vi "Noise Example VISA.vi"() -> ()   [LabVIEW 2012]
doc: "This example demonstrates how to use the various statistics VI's in the Analysis Library to generate common descriptive statistics quantities."
uses:
  <vilib>/Analysis/baseanly.llb/Unimode.vi
  <vilib>/Analysis/NI_AALPro.lvlib
  <vilib>/Analysis/NI_AALBase.lvlib
panel:
  in  "medie":i32=36
  out "Noise 2":dbl[](graph)
  out "Histogram 2":T1(graph)
  out "Mean 2":dbl=0.028574228286743178 format="%.2f"
  out "STD 2":dbl=0.9724758954834173 format="%.2f"
  out "Variance 2":dbl=0.028574228286743168 format="%.2f"
  out "Skewness 2":dbl=0.2146149630445097 format="%.2f"
  out "Kurtosis 2":dbl=2.530711352055369 format="%.2f"
  out "Mode 2":dbl=0.23823547363281233 format="%.2f"
  out "Mode":dbl=0.23823547363281233 format="%.2f"
  out "Kurtosis":dbl=2.530711352055369 format="%.2f"
  out "Skewness":dbl=0.2146149630445097 format="%.2f"
  out "Variance":dbl=0.028574228286743168 format="%.2f"
  out "STD":dbl=0.9724758954834173 format="%.2f"
  out "Mean":dbl=0.028574228286743178 format="%.2f"
  in  "Intervals":i32=100
  in  "Samples":i32=500
  out "Noise":dbl[](graph)
  out "Histogram":T1(graph)
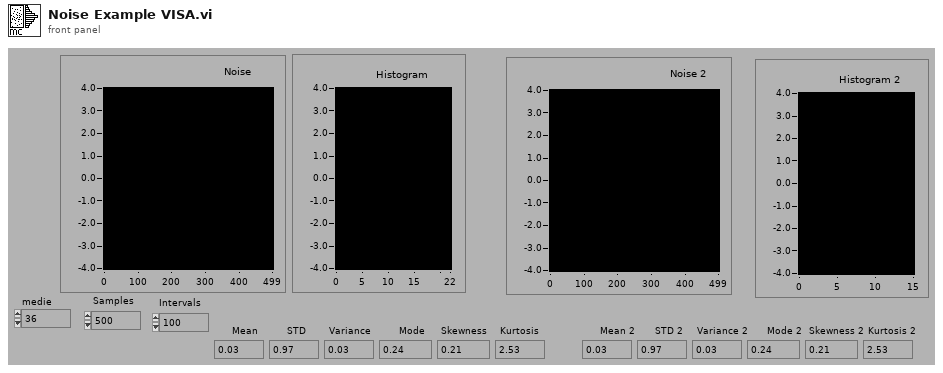
[diagram p1: front panel]
types:
  T1 = cluster{"Histogram: h(x)":i32[], "X Values":dbl[]}
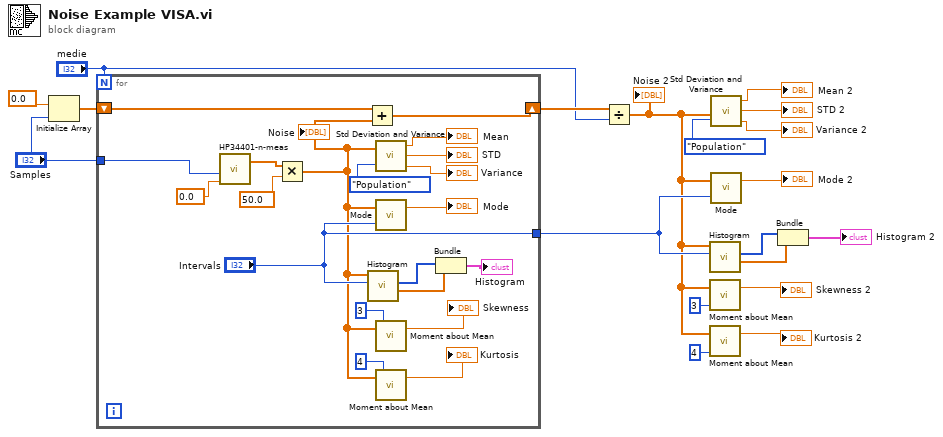
[diagram p0: block diagram]
diagram:
  n1 = Initialize Array(0.0 ("Element Data"), "Samples") -> (w1:dbl[])
  n2 = for {
    N: "medie" -> [_]
    tunnel: ["Intervals"] -> w7
    shift-right: [w26] -> w6
    shift-left: w1 -> [w25]
    tunnel: "Samples" -> [w24]
    n3 = call "HP34401-n-meas.vi"("Tc"=sgl 0.0, "N"=w24) -> ("Vet out"=w21:dbl[])  [unwired: 2 in, 1 out]
    n4 = Multiply(x=w21, y=50.0) -> (x*y=w20:dbl[])
    "Noise" <- w20
    n5 = Add(x=w25, y=w20) -> (x+y=w26:dbl[])
    n6 = call <vilib>:"Histogram.vi"("intervals"="Intervals", "X"=w20) -> ("X Values"=w39:dbl[], "Histogram: h(x)"=w38:i32[])  [unwired: 6 in, 2 out]
    n7 = call <vilib>:"Std Deviation and Variance.vi"("X"=w20, "Weighting (Sample)"=enum16{"Sample", "Population"}."Population") -> ("mean"=→"Mean":dbl, "standard deviation"=→"STD":dbl, "variance"=→"Variance":dbl)
    n8 = call-poly <vilib>:"Mode.vi"("intervals"="Intervals", "X"=w20) -> ("mode"=→"Mode":dbl)  [unwired: 1 out]
    n9 = call <vilib>:"Moment about Mean.vi"("order"=3, "X"=w20) -> ("moment"=→"Skewness":dbl)  [unwired: 1 out]
    n10 = call <vilib>:"Moment about Mean.vi"("order"=4, "X"=w20) -> ("moment"=→"Kurtosis":dbl)  [unwired: 1 out]
    n11 = Bundle("Histogram: h(x)"=w38, "X Values"=w39) -> (→"Histogram":T1)  [unwired: 1 in]
  }
  n12 = Divide(x=w6, y="medie") -> (x/y=w4:dbl[])
  "Noise 2" <- w4
  n13 = call <vilib>:"Histogram.vi"("intervals"=w7, "X"=w4) -> ("X Values"=w8:dbl[], "Histogram: h(x)"=w9:i32[])  [unwired: 6 in, 2 out]
  n14 = call <vilib>:"Moment about Mean.vi"("order"=3, "X"=w4) -> ("moment"=→"Skewness 2":dbl)  [unwired: 1 out]
  n15 = call <vilib>:"Moment about Mean.vi"("order"=4, "X"=w4) -> ("moment"=→"Kurtosis 2":dbl)  [unwired: 1 out]
  n16 = call <vilib>:"Std Deviation and Variance.vi"("X"=w4, "Weighting (Sample)"=enum16{"Sample", "Population"}."Population") -> ("mean"=→"Mean 2":dbl, "standard deviation"=→"STD 2":dbl, "variance"=→"Variance 2":dbl)
  n17 = call-poly <vilib>:"Mode.vi"("intervals"=w7, "X"=w4) -> ("mode"=→"Mode 2":dbl)  [unwired: 1 out]
  n18 = Bundle("Histogram: h(x)"=w9, "X Values"=w8) -> (→"Histogram 2":T1)  [unwired: 1 in]
